vi "ParseSeries.vi"(7 "Series URl":string, 11 "SeriesHTMLBody":string) -> (3 "Series":T1)   [LabVIEW 2022 SP3]
uses:
  TypeDefs/Series.ctl
  <vilib>/Utility/error.llb/Trim Whitespace One-Sided.vi
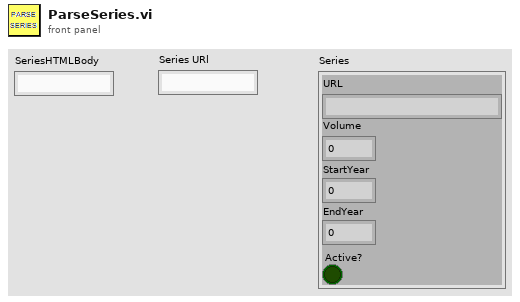
[diagram p1: front panel]
types:
  T1 = typedef "Series.ctl" = cluster{"URL":string, "Volume":i32, "StartYear":i32, "EndYear":i32, "Active?":bool}
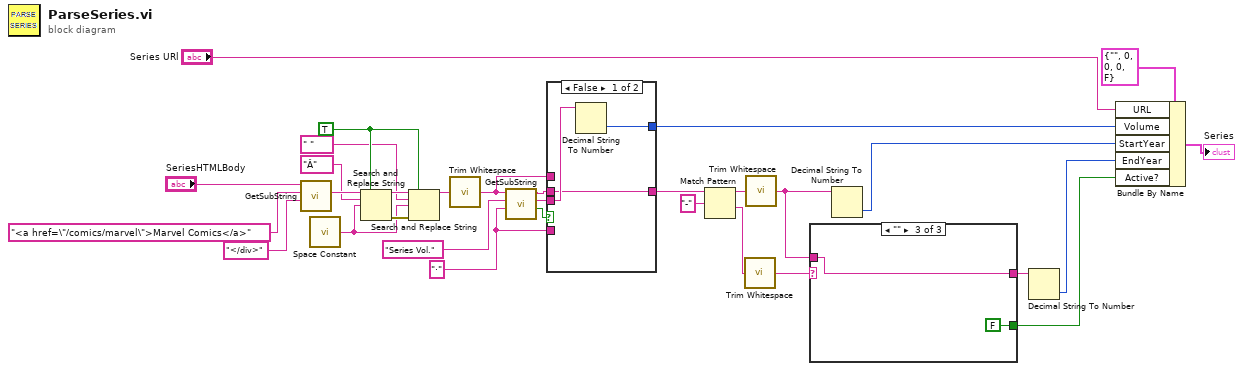
[diagram p0: block diagram]
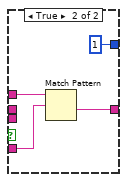
[diagram p2: hidden frame]
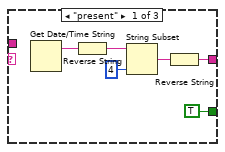
[diagram p3: hidden frame]
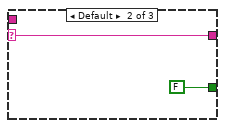
[diagram p4: hidden frame]
diagram:
  w4 = "·" ("End Search")
  w19 = TRUE ("replace all? (F)")
  n1 = call "GetSubString.vi"("End Search"="</div>", "Start Search"="<a href=\"/comics/marvel\">Marvel Comics</a>", "String In"="SeriesHTMLBody") -> ("Match"=w27:string)  [unwired: 6 in, 2 out]
  n2 = call <vilib>:"Space Constant.vi"() -> ("String"=w17:string)
  n3 = Search and Replace String(replace all?=w19, input string=w27, search string="Â" ("End Search"), replace string=w17) -> (result string=w22:string, error out=w21:errorcluster)  [unwired: 4 in, 2 out]
  n4 = Search and Replace String(replace all?=w19, input string=w22, search string=" " ("End Search"), replace string=w17, error in=w21) -> (result string=w20:string)  [unwired: 3 in, 3 out]
  n5 = call <vilib>:"Trim Whitespace.vi"("string"=w20) -> ("trimmed string"=w5:string)  [unwired: 1 in]
  n6 = call "GetSubString.vi"("End Search"=w4, "Start Search"="Series Vol.", "String In"=w5) -> ("Not Found?"=w8:bool, "Match"=w28:string, "Following String Out"=w6:string)  [unwired: 6 in]
  n7 = case shown="False" w8 {
    tunnel: w28 -> [w34 _]
    tunnel: [w33 1] -> w14
    tunnel: [w32 w35] -> w7
    tunnel: w6 -> [w32 _]
    tunnel: w5 -> [_ w37]
    tunnel: w4 -> [_ w36]
    frame False {
      n8 = Decimal String To Number(string=w34) -> (number=w33:i32)  [unwired: 2 in, 1 out]
    }
    frame True {
      n9 = Match Pattern(string=w37, regular expression=w36) -> (after substring=w35:string)  [unwired: 1 in, 3 out]
    }
  }
  n10 = Match Pattern(string=w7, regular expression="-") -> (before substring=w24:string, after substring=w23:string)  [unwired: 1 in, 2 out]
  n11 = call <vilib>:"Trim Whitespace.vi"("string"=w23) -> ("trimmed string"=w16:string)  [unwired: 1 in]
  n12 = call <vilib>:"Trim Whitespace.vi"("string"=w24) -> ("trimmed string"=w9:string)  [unwired: 1 in]
  n13 = case shown="\"\"" w16 {
    selector: w16 -> [_ w46 _]
    tunnel: [w40 w46 w48] -> w15
    tunnel: [TRUE FALSE FALSE] -> w11
    tunnel: w9 -> [_ _ w48]
    frame "present" {
      n14 = Get Date/Time String() -> (date string=w42:string)  [unwired: 3 in, 1 out]
      n15 = Reverse String(1:w42) -> (0:w43:string)
      n16 = String Subset(string=w43, length (rest)=4 ("length (rest)")) -> (substring=w44:string)  [unwired: 1 in]
      n17 = Reverse String(1:w44) -> (0:w40:string)
    }
    frame Default {
    }
    frame "" {
    }
  }
  n18 = Decimal String To Number(string=w9) -> (number=w13:i32)  [unwired: 2 in, 1 out]
  n19 = Decimal String To Number(string=w15) -> (number=w12:i32)  [unwired: 2 in, 1 out]
  n20 = Bundle By Name(cluster=T1 {"URL"="", "Volume"=0, "StartYear"=0, "EndYear"=0, "Active?"=FALSE} ("Series In"), "URL"="Series URl", "Volume"=w14, "StartYear"=w13, "EndYear"=w12, "Active?"=w11) -> (→"Series":T1)
